vi "Get Stream.vi"() -> (0 "Good Data":bool, 1 "UART Stream 2":u8[](array[numeric]))   [LabVIEW 2010]
uses:
  Main Global.vi
panel:
  out "Buffer Dump Size":u32
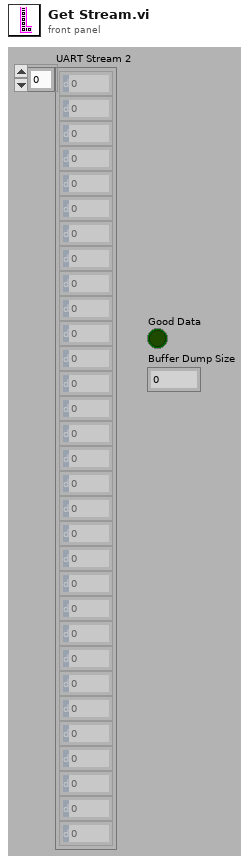
[diagram p1: front panel]
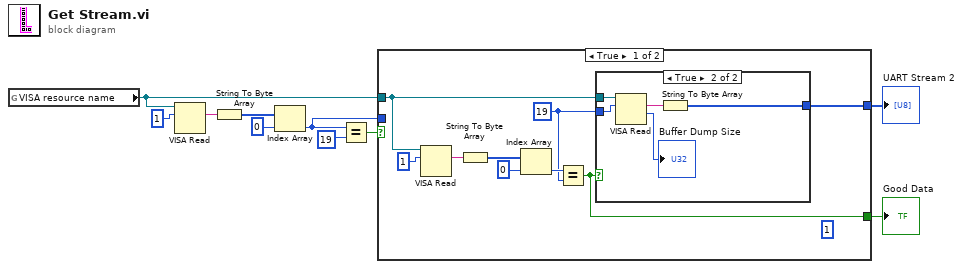
[diagram p0: block diagram]
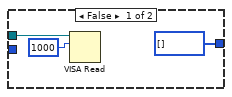
[diagram p2: hidden frame]
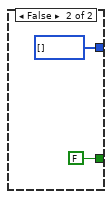
[diagram p3: hidden frame]
diagram:
  n1 = global read "Main Global.vi" "VISA resource name"() -> (w5:refnum<visa-resource-name>)
  n2 = VISA Read(VISA resource name=w5, byte count=u32 1) -> (read buffer=w4:string)  [unwired: 1 in, 3 out]
  n3 = String To Byte Array(string=w4) -> (unsigned byte array=w3:u8[])
  n4 = Index Array(array=w3, index=0) -> (element=w6:u8)
  n5 = Equal?(x=w6, y=u8 19) -> (x = y?=w9:bool)
  n6 = case shown="True" w9 {
    tunnel: w6 -> [_ _]
    tunnel: w5 -> [w14 _]
    tunnel: [w12 u8[] [] ("unsigned byte array")] -> w2
    tunnel: [w11 FALSE] -> w1
    frame True {
      w13 = u8 19 ("y")
      (unwired) 1 ("index")
      n7 = VISA Read(VISA resource name=w14, byte count=u32 1) -> (read buffer=w18:string)  [unwired: 1 in, 3 out]
      n8 = String To Byte Array(string=w18) -> (unsigned byte array=w17:u8[])
      n9 = Index Array(array=w17, index=0) -> (element=w15:u8)
      n10 = Equal?(x=w15, y=w13) -> (x = y?=w11:bool)
      n11 = case shown="True" w11 {
        tunnel: w14 -> [w21 w27]
        tunnel: w13 -> [_ w26]
        tunnel: [u8[] [] ("unsigned byte array") w24] -> w12
        frame False {
          n12 = VISA Read(VISA resource name=w21, byte count=u32 1000) -> ()  [unwired: 1 in, 4 out]
        }
        frame True {
          n13 = VISA Read(VISA resource name=w27, byte count=w26) -> (read buffer=w25:string, return count=→"Buffer Dump Size":u32)  [unwired: 1 in, 2 out]
          n14 = String To Byte Array(string=w25) -> (unsigned byte array=w24:u8[])
        }
      }
    }
    frame False {
    }
  }
  "UART Stream 2" <- w2
  "Good Data" <- w1
